vi "Test Configuration.vi"(8 "error in (no error)":errorcluster, 11 "Settings in":T1) -> (0 "error out":errorcluster, 2 "all rows":string[][](array[string]), 3 "output cluster":T1)   [LabVIEW 2026]
uses:
  Settings/Settings.ctl
  Acquisition/Hardware Configuration.ctl
  Logging/Logging Configuration.ctl
  <vilib>/Utility/config.llb/Read Key (String).vi
  <vilib>/Utility/config.llb/NI_LVConfig.lvlib
  Acquisition/Acquisition.lvlib
  Logging/Logging.lvlib
  Settings/Settings.lvlib
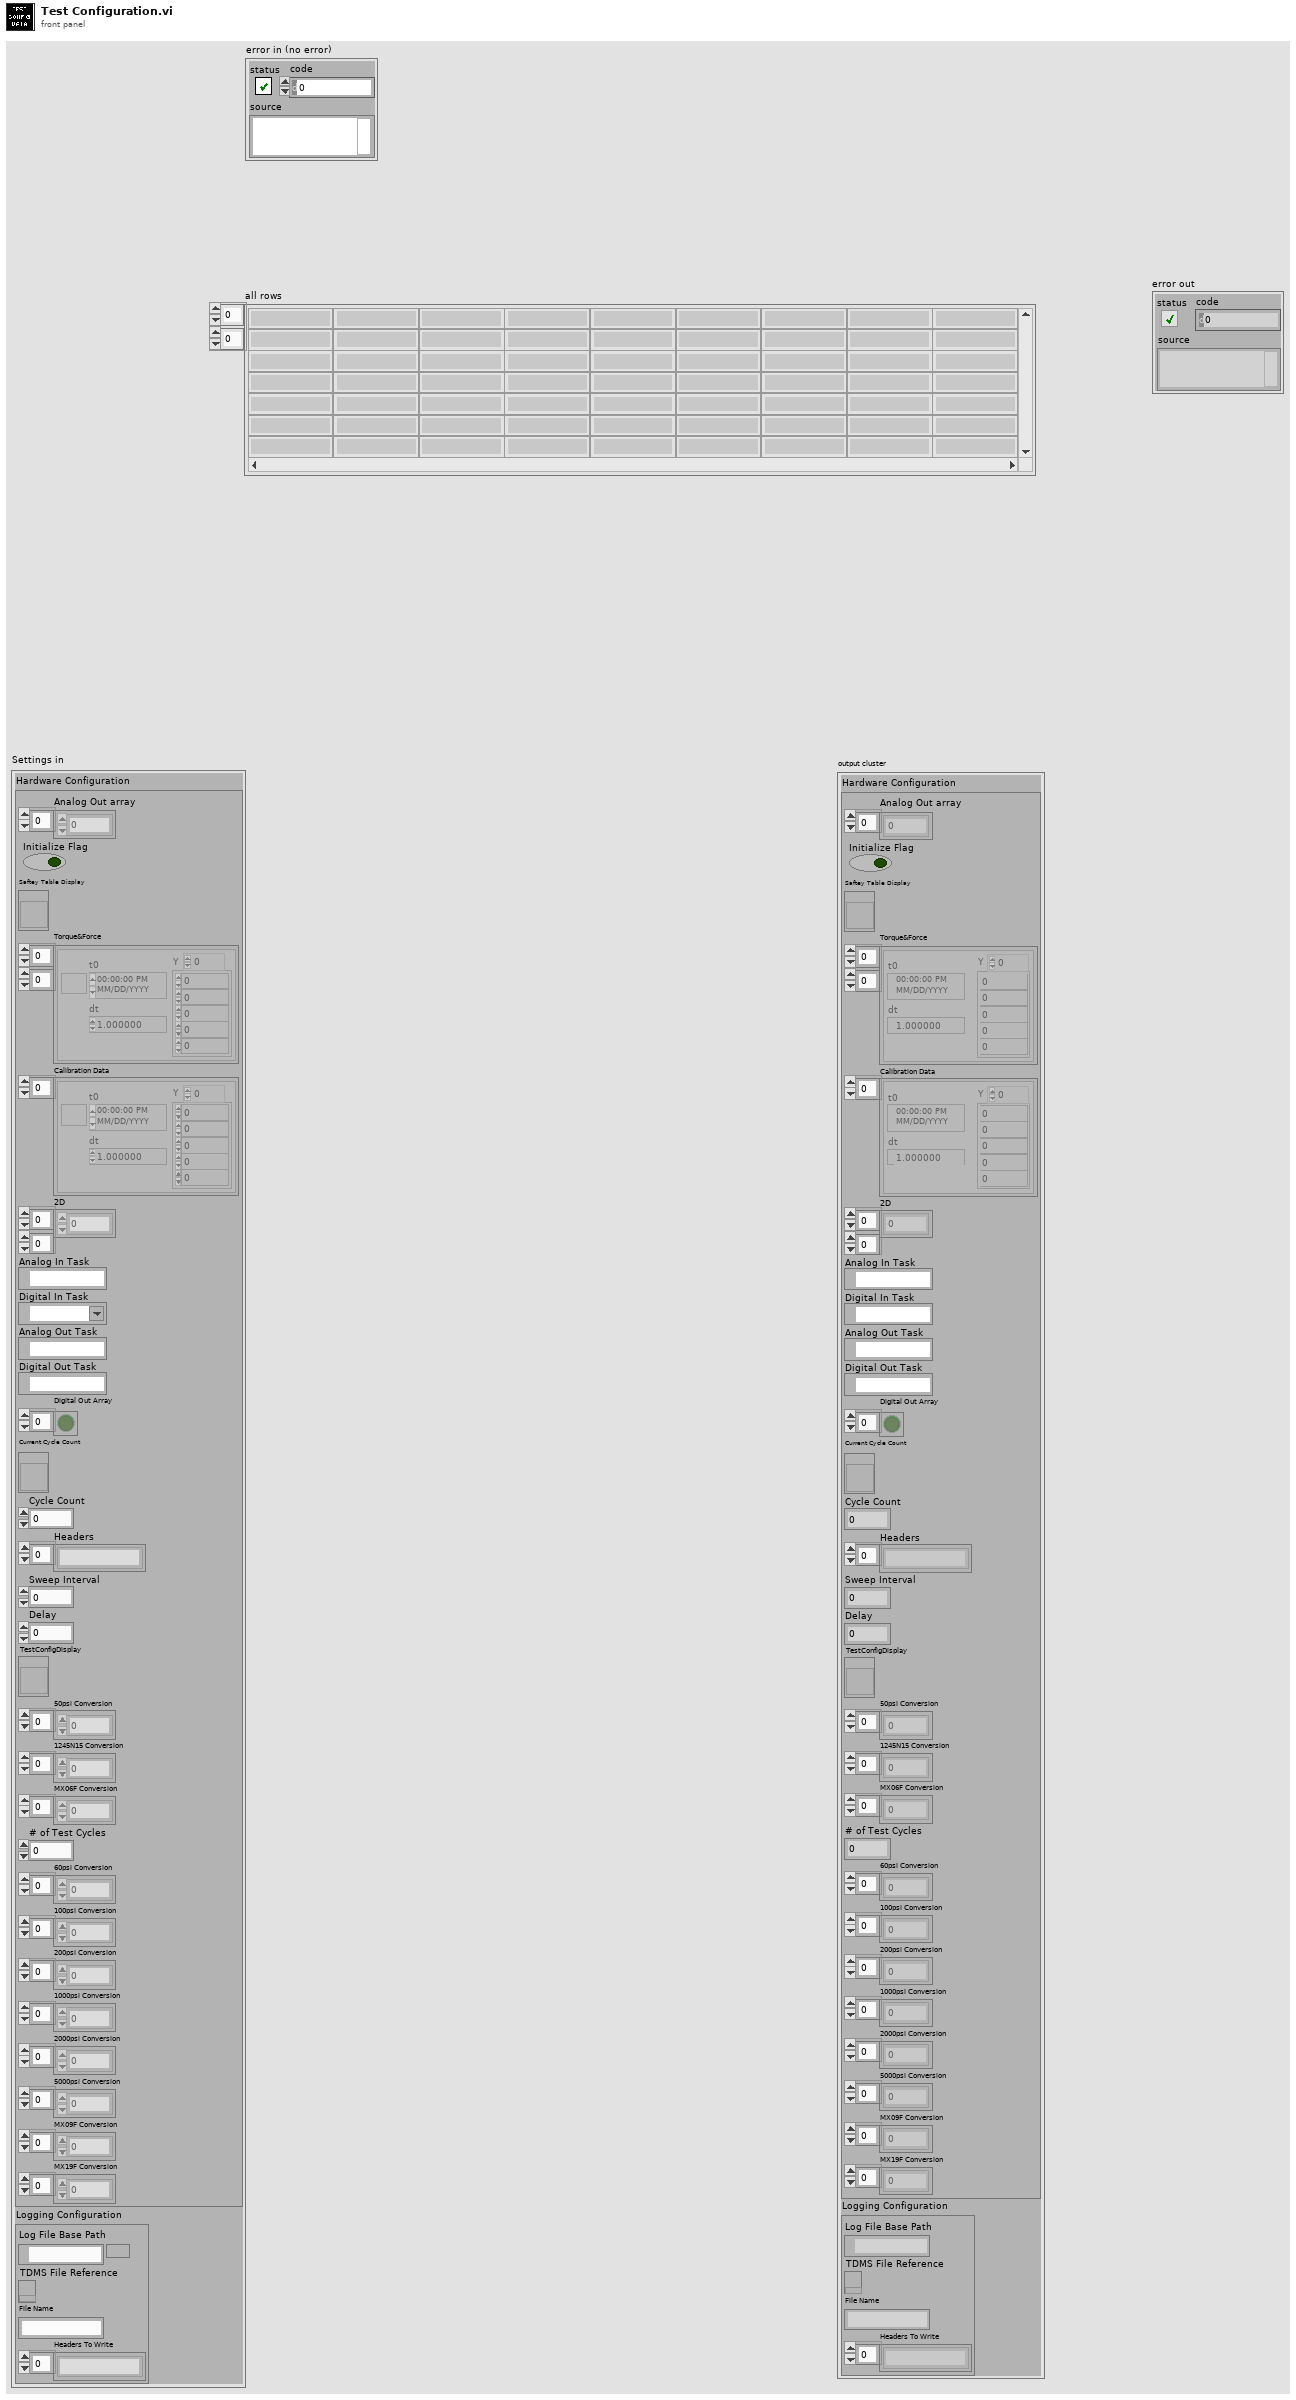
[diagram p1: front panel]
types:
  T1 = typedef "Settings.lvlib/Settings.ctl" = cluster{"Hardware Configuration":T2, "Logging Configuration":T3}
  T2 = typedef "Acquisition.lvlib/Hardware Configuration.ctl" = cluster{"Analog Out array":dbl[], "Initialize Flag":bool, "Saftey Table Display":refnum<vi>, "Torque&Force":waveform(dbl)[][], "Calibration Data":waveform(dbl)[], "2D":dbl[][], "Analog In Task":refnum<k21>, "Digital In Task":refnum<k21>, "Analog Out Task":refnum<k21>, "Digital Out Task":refnum<k21>, "Digital Out Array":bool[], "Current Cycle Count":refnum<vi>, "Cycle Count":u64, "Headers":string[], "Sweep Interval":u64, "Delay":u64, "TestConfigDisplay":refnum<vi>, "50psi Conversion":dbl[], "1245N15 Conversion":dbl[], "MX06F Conversion":dbl[], "# of Test Cycles":u64, "60psi Conversion":dbl[], "100psi Conversion":dbl[], "200psi Conversion":dbl[], "1000psi Conversion":dbl[], "2000psi Conversion":dbl[], "5000psi Conversion":dbl[], "MX09F Conversion":dbl[], "MX19F Conversion":dbl[]}
  T3 = typedef "Logging.lvlib/Logging Configuration.ctl" = cluster{"Log File Base Path":path, "TDMS File Reference":refnum<k34>, "File Name":string, "Headers To Write":string[]}
  T4 = typedef "NI_LVConfig.lvlib/Config Data RefNum.ctl" = refnum<k1>
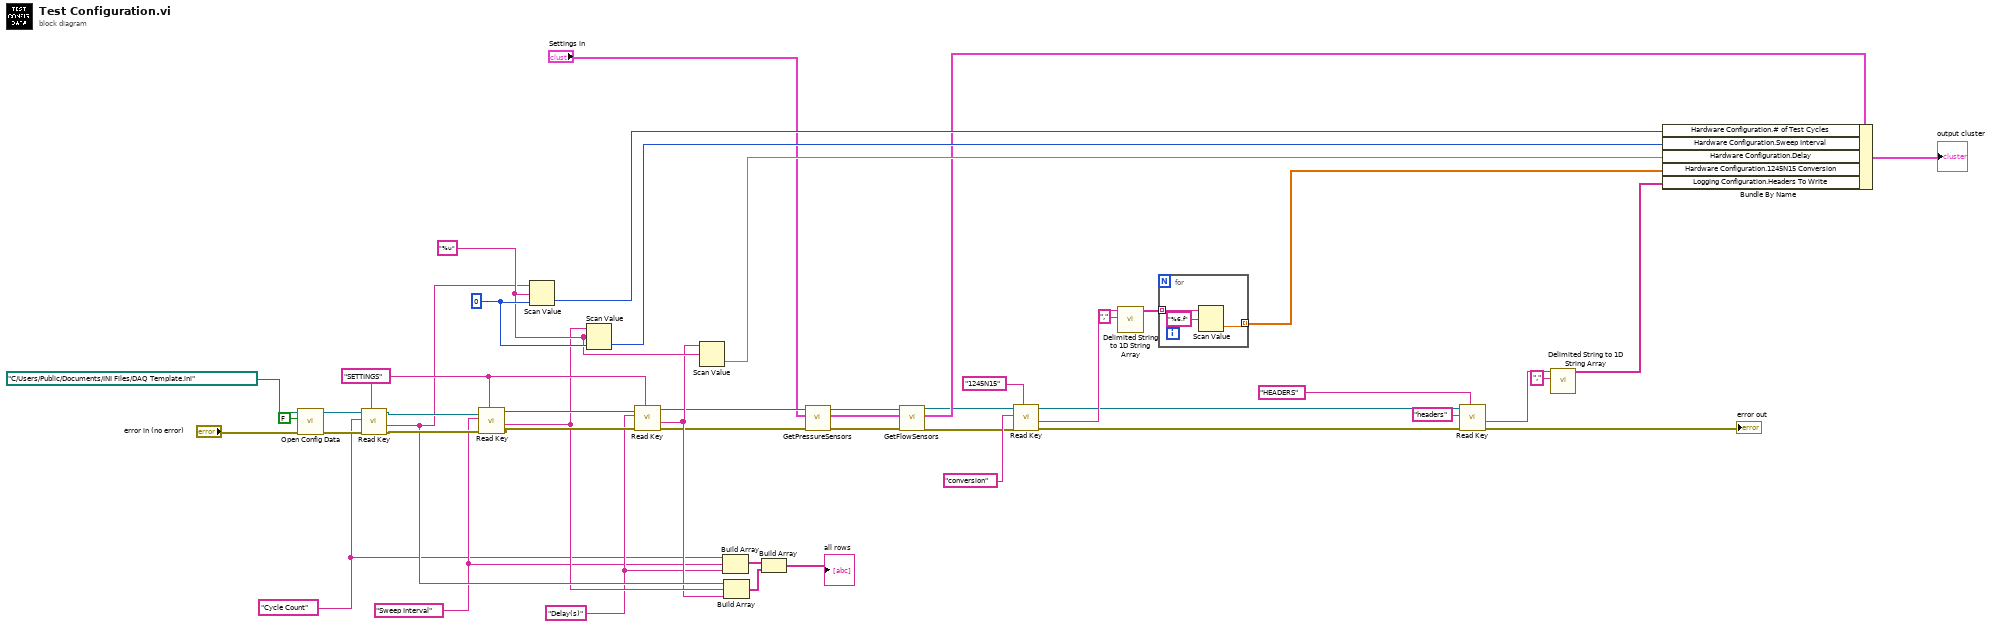
[diagram p0: block diagram]
diagram:
  w39 = "%u" ("format string")
  w42 = u64 0
  w19 = "Delay(s)" ("key")
  w18 = "Sweep Interval" ("key")
  w26 = "SETTINGS" ("section")
  w17 = "Cycle Count" ("key")
  n1 = call <vilib>:"Open Config Data.vi"("error in (no error)"="error in (no error)", "create file if necessary (T)"=FALSE, "configuration file path"=path "C:/Users/Public/Documents/INI Files/DAQ Template.ini") -> ("error out"=w48:errorcluster, "refnum"=w16:T4)  [unwired: 6 in, 1 out]
  n2 = call-poly <vilib>:"Read Key.vi"("section"=w26, "error in (no error)"=w48, "key"=w17, "refnum"=w16) -> ("error out"=w46:errorcluster, "value"=w24:string, "refnum out"=w47:T4)  [unwired: 4 in, 1 out]
  n3 = call-poly <vilib>:"Read Key.vi"("section"=w26, "error in (no error)"=w46, "key"=w18, "refnum"=w47) -> ("error out"=w45:errorcluster, "value"=w23:string, "refnum out"=w44:T4)  [unwired: 4 in, 1 out]
  n4 = Scan Value(string=w24, format string=w39, default (0 dbl)=w42) -> (value=w43:u64)  [unwired: 1 out]
  n5 = Scan Value(string=w23, format string=w39, default (0 dbl)=w42) -> (value=w41:u64)  [unwired: 1 out]
  n6 = call-poly <vilib>:"Read Key.vi"("section"=w26, "error in (no error)"=w45, "key"=w19, "refnum"=w44) -> ("error out"=w11:errorcluster, "value"=w22:string, "refnum out"=w10:T4)  [unwired: 4 in, 1 out]
  n7 = Scan Value(string=w22, format string=w39) -> (value=w40:dbl)  [unwired: 1 in, 1 out]
  n8 = Build Array(w17, w18, w19) -> (w20:string[])
  n9 = Build Array(w24, w23, w22) -> (w25:string[])
  n10 = Build Array(w20, w25) -> (→"all rows":string[][])
  n11 = call "GetPressureSensors.vi"("error in (no error)"=w11, "Settings in"="Settings in", "refnum"=w10) -> ("error out"=w5:errorcluster, "Settings out"=w4:T1, "refnum out"=w6:T4)  [unwired: 6 in]
  n12 = call "GetFlowSensors.vi"("error in (no error)"=w5, "Settings in"=w4, "refnum"=w6) -> ("error out"=w1:errorcluster, "Settings out"=w3:T1, "refnum out"=w2:T4)  [unwired: 6 in]
  n13 = call-poly <vilib>:"Read Key.vi"("section"="1245N15", "error in (no error)"=w1, "key"="conversion", "refnum"=w2) -> ("error out"=w7:errorcluster, "value"=w36:string, "refnum out"=w8:T4)  [unwired: 4 in, 1 out]
  n14 = call <vilib>:"Delimited String to 1D String Array.vi"("delimiter"=",", "delimited string"=w36) -> ("string array"=w37:string[])  [unwired: 9 in]
  n15 = for {
    tunnel: w37 -> [w51] mode=indexing
    tunnel: [w49] -> w34 mode=indexing
    n16 = Scan Value(string=w51, format string="%6.f") -> (value=w49:dbl)  [unwired: 1 in, 1 out]
  }
  n17 = call-poly <vilib>:"Read Key.vi"("section"="HEADERS", "error in (no error)"=w7, "key"="headers", "refnum"=w8) -> ("error out"=→"error out":errorcluster, "value"=w30:string)  [unwired: 4 in, 2 out]
  n18 = call <vilib>:"Delimited String to 1D String Array.vi"("delimiter"=",", "delimited string"=w30) -> ("string array"=w27:string[])  [unwired: 9 in]
  n19 = Bundle By Name(cluster=w3, "Hardware Configuration.# of Test Cycles"=w43, "Hardware Configuration.Sweep Interval"=w41, "Hardware Configuration.Delay"=w40, "Hardware Configuration.1245N15 Conversion"=w34, "Logging Configuration.Headers To Write"=w27) -> (→"output cluster":T1)
